vi "process_probe_resistance_array.vi"(8 "error in (no error)":errorcluster, 11 "TempProbe in":refnum<class "TempProbe.lvclass">) -> (0 "error out":errorcluster, 1 "resistance average":dbl, 2 "temperature":dbl, 3 "TempProbe out":refnum<class "TempProbe.lvclass">, 4 "resistance standard deviation":dbl)   [LabVIEW 2010, in "TempProbe.lvclass"]
uses:
  TempProbe.lvclass
  accessors/read_r_to_t_equation.vi
  accessors/read_resistances_array_from_probe.vi
  <vilib>/Analysis/NI_AALBase.lvlib
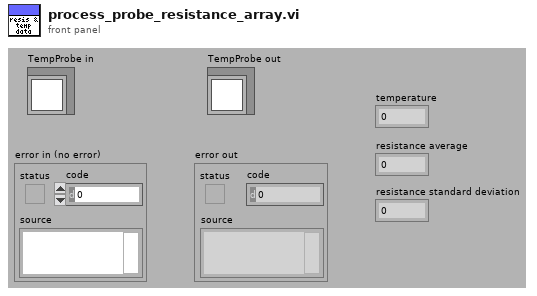
[diagram p1: front panel]
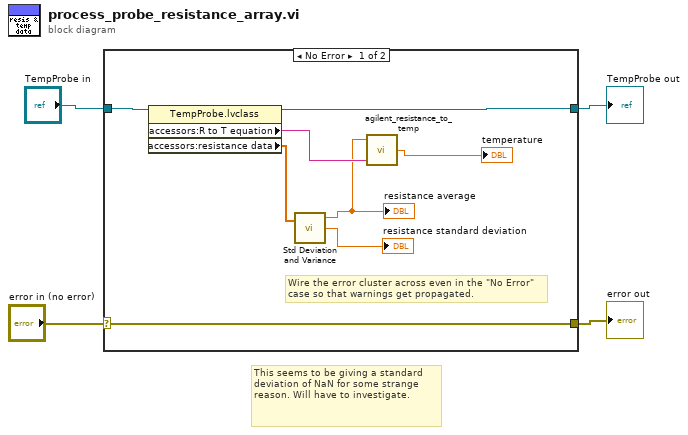
[diagram p0: block diagram]
diagram:
  # "This seems to be giving a standard deviation of NaN for some strange reason. Will have to investigate."
  n1 = case shown="No Error" "error in (no error)" {
    selector: "error in (no error)" -> [w11 w14]
    tunnel: [w11 w14] -> w3
    tunnel: [w9 w13] -> w1
    tunnel: "TempProbe in" -> [w12 w13]
    frame No Error {
      # "Wire the error cluster across even in the \"No Error\"\ncase so that warnings get propagated."
      n2 = property class="TempProbe.lvclass"(reference=w12) -> (reference out=w9:refnum<class "TempProbe.lvclass">, "accessors:R to T equation"=w7:string, "accessors:resistance data"=w8:dbl[])  [unwired: 1 in, 1 out]
      n3 = call <vilib>:"Std Deviation and Variance.vi"("X"=w8) -> ("mean"=w6:dbl, "standard deviation"=→"resistance standard deviation":dbl)  [unwired: 1 in, 1 out]
      "resistance average" <- w6
      n4 = call "agilent_resistance_to_temp.vi"("T equation"=w7, "Resistance"=w6) -> ("Temperature"=→"temperature":dbl)  [unwired: 1 in]
    }
    frame Error {
    }
  }
  "error out" <- w3
  "TempProbe out" <- w1
